vi "sv_UFF58 Check Data Valid (Freq - Complex) (N Ch).vi"(5 "real part in":cluster{"f0":dbl, "df":dbl, "magnitude":dbl[]}[](array[cluster]) {"magnitude" format="%.2p"; "df" format="%.2p"; "f0" format="%.2p"}, 7 "imaginary part in":cluster{"f0":dbl, "df":dbl, "magnitude":dbl[]}[](array[cluster]) {"magnitude" format="%.2p"; "df" format="%.2p"; "f0" format="%.2p"}, 9 "spectrum info in":T1[](array[typedef]) {"x-axis units" items=["Time (s)"=0, "Frequency-CB (Hz)"=1, "Frequency-CPB (Hz)"=1248, "Frequency-Arbitrary (Hz)"=2357, "Quefrency (s)"=2, "Revolutions (rev)"=3, "Order"=4, "Speed (RPM)"=11, "Speed (rad/s)"=21, "Index"=65535]; "weighting filter" items=["Linear", "A-weighting", "B-weighting", "C-weighting", "ITU-R 468-4", "Dolby", "CCITT", "C-message", "Wb", "Wc", "Wd", "We", "Wf", "Wh", "Wj", "Wk", "Wm", "AES17 20 kHz lowpass", "AES17 40 kHz lowpass", "AES17 20 kHz highpass", "AES17 40 kHz highpass"]; "dB reference [EU]" format="%.2f"; "engineering units" items=["custom..."=0, "V"=1, "A"=21, "C"=30, "pC"=31, "s"=32, "-"=29, "Pa"=2, "N"=20, "g"=3, "m/s^2"=4, "m/s"=5, "m"=6, "mm/s"=12, "mm"=13, "micron/s"=14, "micron"=15, "in/s^2"=7, "in/s"=8, "in"=9, "mil/s"=10, "mil"=11, "rad/s^2"=16, "rad/s"=17, "rad"=18, "deg/s^2"=26, "deg/s"=27, "deg"=28, "RPM"=22, "cycle/s^2"=23, "Hz"=24, "cycle"=25, "strain"=19]; "spectral info"."window" items=["None "=0, "Hanning"=1, "Hamming"=2, "Blackman-Harris"=3, "Exact Blackman"=4, "Blackman"=5, "Flat Top"=6, "4 Term B-Harris "=7, "7 Term B-Harris"=8, "Low Sidelobe"=9, "Force - Exponential"=10, "Gaussian"=62]}, 11 "error in (no error)":errorcluster) -> (6 "real part out":cluster{"f0":dbl, "df":dbl, "magnitude":dbl[]}[](array[cluster]) {"magnitude" format="%.2p"; "df" format="%.2p"; "f0" format="%.2p"}, 8 "imaginary part out":cluster{"f0":dbl, "df":dbl, "magnitude":dbl[]}[](array[cluster]) {"magnitude" format="%.2p"; "df" format="%.2p"; "f0" format="%.2p"}, 10 "spectrum info out":T1[](array[typedef]) {"x-axis units" items=["Time (s)"=0, "Frequency-CB (Hz)"=1, "Frequency-CPB (Hz)"=1248, "Frequency-Arbitrary (Hz)"=2357, "Quefrency (s)"=2, "Revolutions (rev)"=3, "Order"=4, "Speed (RPM)"=11, "Speed (rad/s)"=21, "Index"=65535]; "weighting filter" items=["Linear", "A-weighting", "B-weighting", "C-weighting", "ITU-R 468-4", "Dolby", "CCITT", "C-message", "Wb", "Wc", "Wd", "We", "Wf", "Wh", "Wj", "Wk", "Wm", "AES17 20 kHz lowpass", "AES17 40 kHz lowpass", "AES17 20 kHz highpass", "AES17 40 kHz highpass"]; "dB reference [EU]" format="%.2f"; "engineering units" items=["custom..."=0, "V"=1, "A"=21, "C"=30, "pC"=31, "s"=32, "-"=29, "Pa"=2, "N"=20, "g"=3, "m/s^2"=4, "m/s"=5, "m"=6, "mm/s"=12, "mm"=13, "micron/s"=14, "micron"=15, "in/s^2"=7, "in/s"=8, "in"=9, "mil/s"=10, "mil"=11, "rad/s^2"=16, "rad/s"=17, "rad"=18, "deg/s^2"=26, "deg/s"=27, "deg"=28, "RPM"=22, "cycle/s^2"=23, "Hz"=24, "cycle"=25, "strain"=19]; "spectral info"."window" items=["None "=0, "Hanning"=1, "Hamming"=2, "Blackman-Harris"=3, "Exact Blackman"=4, "Blackman"=5, "Flat Top"=6, "4 Term B-Harris "=7, "7 Term B-Harris"=8, "Low Sidelobe"=9, "Force - Exponential"=10, "Gaussian"=62]}, 15 "error out":errorcluster)   [LabVIEW 2017, in "SoundVib_UFF58.lvlib"]
uses:
  <vilib>/addons/Sound and Vibration/svt_UFF58/SoundVib_UFF58.lvlib
  <vilib>/addons/_NISVFA/_Shared subVIs/Controls/svc_Spectrum Info.ctl
  <vilib>/addons/_NISVFA/_Shared subVIs/Controls/svc_X-Axis Units.ctl
  <vilib>/addons/_NISVFA/_Shared subVIs/Controls/svc_Spectrum Type.ctl
  <vilib>/addons/_NISVFA/_Shared subVIs/Controls/svc_Engineering Units Text Ring.ctl
  <vilib>/addons/_NISVFA/_Shared subVIs/Controls/svc_Weighting Filter Text Ring.ctl
  <vilib>/addons/_NISVFA/_Shared subVIs/Controls/svc_Complimentary Spectrum Units.ctl
  <vilib>/addons/_NISVFA/_Spectrum Processing/SVFA Magnitude and Phase to Real and Imaginary (N Ch).vi
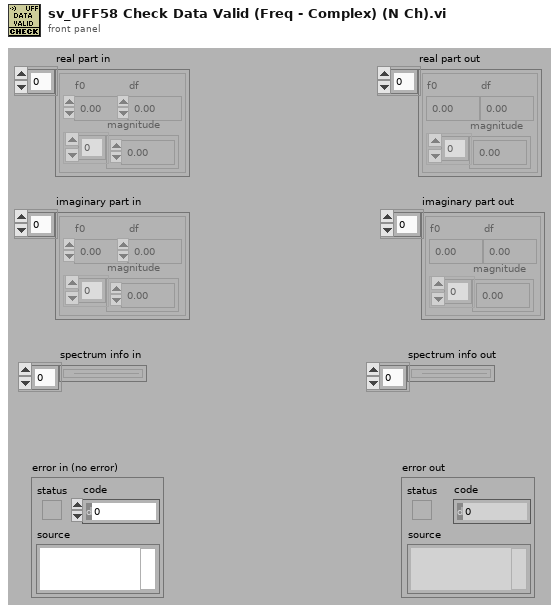
[diagram p1: front panel]
types:
  T1 = typedef "svc_Spectrum Info.ctl" = cluster{"channel name":string, "description":string, "x-axis units":T2, "spectral info":cluster{"spectrum type":T3, "linear/dB":enum16{"linear", "dB"}, "window":u16, "window size":i32, "FFT size":i32}, "engineering units":T4, "custom label":string, "dB reference [EU]":dbl, "peak units":enum16{"rms", "peak", "peak-peak"}, "weighting filter":T5, "spectral density?":bool, "unit label":string, "spectrum skewed?":bool, "complimentary spectrum units":T6}
  T2 = typedef "svc_X-Axis Units.ctl" = u16
  T3 = typedef "svc_Spectrum Type.ctl" = enum16{"FFT Spectrum [complex]", "Amplitude [Magnitude]", "Power [Magnitude^2]", "Cross Spectrum [complex]", "Frequency Response [Complex]"}
  T4 = typedef "svc_Engineering Units Text Ring.ctl" = u16
  T5 = typedef "svc_Weighting Filter Text Ring.ctl" = u16
  T6 = typedef "svc_Complimentary Spectrum Units.ctl" = enum16{"none", "radians", "degrees", "cycles", "imaginary"}
  T7 = cluster{"x0":dbl, "dx":dbl, "imaginary part":dbl[]}[]
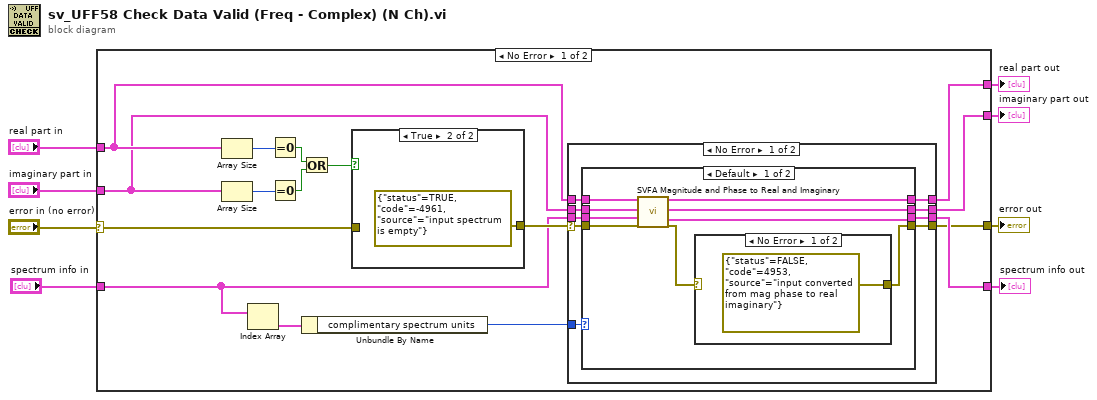
[diagram p0: block diagram]
diagram:
  n1 = case shown="No Error" "error in (no error)" {
    selector: "error in (no error)" -> [w24 w58]
    tunnel: "real part in" -> [w17 w57]
    tunnel: [w12 w58] -> w8
    tunnel: [w16 w57] -> w5
    tunnel: "imaginary part in" -> [w15 w56]
    tunnel: [w14 w56] -> w3
    tunnel: "spectrum info in" -> [w11 w55]
    tunnel: [w13 w55] -> w1
    frame No Error {
      n2 = Array Size(array=w17) -> (size(s)=w23:i32)
      n3 = Array Size(array=w15) -> (size(s)=w22:i32)
      n4 = Index Array(array=w11) -> (element=w10:T1)  [unwired: 1 in]
      n5 = Equal To 0?(x=w23) -> (x = 0?=w21:bool)
      n6 = Equal To 0?(x=w22) -> (x = 0?=w20:bool)
      n7 = Or(x=w21, y=w20) -> (x .or. y?=w19:bool)
      n8 = Unbundle By Name(w10) -> ("complimentary spectrum units"=w9:T6)
      n9 = case shown="True" w19 {
        tunnel: w24 -> [w53 _]
        tunnel: [w53 errorcluster {"status"=TRUE, "code"=-4961, "source"="input spectrum is empty"} ("error IO")] -> w18
        frame False {
        }
        frame True {
        }
      }
      n10 = case shown="No Error" w18 {
        selector: w18 -> [w31 w52]
        tunnel: [w32 w52] -> w12
        tunnel: w9 -> [w33 _]
        tunnel: w17 -> [w30 w51]
        tunnel: w15 -> [w29 w50]
        tunnel: w11 -> [w28 w49]
        tunnel: [w27 w51] -> w16
        tunnel: [w26 w50] -> w14
        tunnel: [w25 w49] -> w13
        frame No Error {
          n11 = case shown="Default" w33 {
            tunnel: [w35 w48] -> w32
            tunnel: w31 -> [w42 w48]
            tunnel: w30 -> [w41 w47]
            tunnel: w29 -> [w40 w46]
            tunnel: w28 -> [w39 w45]
            tunnel: [w38 w47] -> w27
            tunnel: [w37 w46] -> w26
            tunnel: [w36 w45] -> w25
            frame Default {
              n12 = call-poly <vilib>:"SVFA Magnitude and Phase to Real and Imaginary.vi"("magnitude spectra"=w41, "phase spectra"=w40, "spectrum info in"=w39, "error in (no error)"=w42) -> ("real spectra"=w38:cluster{"x0":dbl, "dx":dbl, "real part":dbl[]}[], "imaginary spectra"=w37:T7, "spectrum info out"=w36:T1[], "error out"=w34:errorcluster)  [unwired: 10 in, 2 out]
              n13 = case shown="No Error" w34 {
                selector: w34 -> [_ w44]
                tunnel: [errorcluster {"status"=FALSE, "code"=4953, "source"="input converted from mag phase to real imaginary"} ("error IO") w44] -> w35
                frame No Error {
                }
                frame Error {
                }
              }
            }
            frame "imaginary" {
            }
          }
        }
        frame Error {
        }
      }
    }
    frame Error {
    }
  }
  "error out" <- w8
  "real part out" <- w5
  "imaginary part out" <- w3
  "spectrum info out" <- w1
